vi "Mutual_Info_Score.vi"(8 "error in (no error)":errorcluster caption="entrée d'erreur (pas d'erreur)", 9 "labels_pred":string[][](array[string]), 10 "labels_true":string[][](array[string]), 11 "mutual_info_score":T1) -> (0 "error out":errorcluster caption="sortie d'erreur", 3 "Score":string)   [LabVIEW 2020]
doc: "Mutual Information between two clusterings.\n\nThe Mutual Information is a measure of the similarity between two labels of the same data.\n\nThis metric is independent of the absolute values of the labels: a permutation of the class or cluster label values won’t change the score value in any way.\n\nThis metric is furthermore symmetric: switching label_true with label_pred will return the same score value. This can be useful to measure the agreement of two independent label assignments strategies on the same dataset when the real ground truth is not known.\n\n\nParameters : \n\n- labels_true : int array, shape = [n_samples]\nA clustering of the data into disjoint subsets.\n\n- labels_pred : int array-like of shape (n_samples,)\nA clustering of the data into disjoint subsets.\n\n- contingency : {None, array, sparse matrix}, shape = [n_classes_true, n_classes_pred]\nA contingency matrix given by the contingency_matrix function. If value is None, it will be computed, otherwise the given value is used, with labels_true and labels_pred ignored.\n\nReturns : \n\n- mi : float\nMutual information, a non-negative value"
uses:
  Mutual_Info_Score.lvclass
panel:
  out "Mutual_Info_Score.lvclass":refnum<class "Mutual_Info_Score.lvclass">
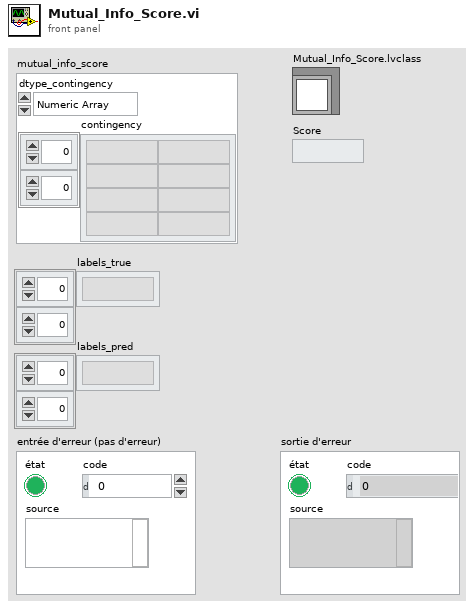
[diagram p1: front panel]
types:
  T1 = cluster{"dtype_contingency":enum16{"Numeric Array", "String Array", "Sparse"}, "contingency":string[][]}
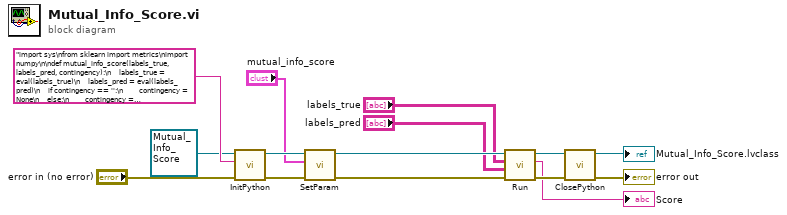
[diagram p0: block diagram]
diagram:
  n1 = call-dynamic "InitPython.vi"("error in (no error)"="error in (no error)", "Python Instruction"="import sys\nfrom sklearn import metrics\nimport numpy\n\ndef mutual_info_score(labels_true, labels_pred, contingency):\n    labels_true = eval(labels_true)\n    labels_pred = eval(labels_pred)\n    if contingency == '':\n        contingency = None\n    else:\n        contingency = eval(contingency)\n    try:\n        mutual_info_score = metrics.mutual_info_score(labels_true, labels_pred, contingency)\n        mutual_info_score = mutual_info_score.tolist()\n        return str(mutual_info_score)\n    except:\n        erreur = sys.exc_info()\n        typerr = u\"%s\" % (erreur[0])\n        typerr = typerr[typerr.find(\"'\")+1:typerr.rfind(\"'\")]\n        msgerr = u\"%s\" % (erreur[1])\n        message = str('/!\\\\ {0} : {1}'. format(typerr,msgerr))\n        return message", "Scikit-learn en entrée"=refnum<class "Mutual_Info_Score.lvclass"> refnum ("Mutual_Info_Score.lvclass")) -> ("error out"=w11:errorcluster, "Scikit-learn en sortie"=w10:refnum<class "Mutual_Info_Score.lvclass">)  [unwired: 7 in]
  n2 = call-dynamic "SetParam.vi"("error in (no error)"=w11, "mutual_info_score"="mutual_info_score", "Mutual_Info_Score.lvclass"=w10) -> ("error out"=w8:errorcluster, "Mutual_Info_Score.lvclass"=w9:refnum<class "Mutual_Info_Score.lvclass">)  [unwired: 7 in]
  n3 = call-dynamic "Run.vi"("error in (no error)"=w8, "labels_pred"="labels_pred", "labels_true"="labels_true", "Mutual_Info_Score.lvclass"=w9) -> ("error out"=w6:errorcluster, "String Data"=→"Score":string, "Mutual_Info_Score.lvclass"=w7:refnum<class "Mutual_Info_Score.lvclass">)  [unwired: 5 in]
  n4 = call-dynamic "ClosePython.vi"("error in (no error)"=w6, "Scikit-learn en entrée"=w7) -> ("error out"=→"error out":errorcluster, "Scikit-learn en sortie"=→"Mutual_Info_Score.lvclass":refnum<class "Mutual_Info_Score.lvclass">)  [unwired: 8 in]
